vi "Log_ADAM_scan_table.vi"() -> ()   [LabVIEW 2022 SP3]
uses:
  ADAM Client/Sub VIs/ADAM Controls/Channel_State.ctl
  Anemometry/Anemometry Sub Vis/Globals/Constants_global.vi
  Anemometry/Anemometry Sub Vis/Globals/Preference_global.vi
  ADAM_Global.vi
  Anemometry/Anemometry Sub Vis/Globals/Meas_global.vi
  ADAM Client/Sub VIs/Channel_State_Control.ctl
panel:
  in  "Averaging time (Seconds)":dbl=60.0
  out "Current time":string
  out "Started Time":string
  in  "stop":bool
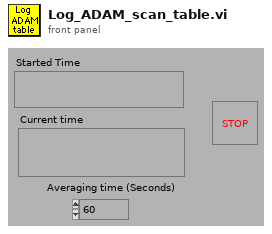
[diagram p1: front panel]
types:
  T1 = enum16{"On", "Off", "Always On", "Always Off", "Delete"}
  T2 = enum16{"Load ADAM setup from excel file", "Save ADAM setup to excel file"}
  T3 = typedef "Channel_State_Control.ctl" = enum16{"Channel Name", "Channel Name Starts with", "Main Address"}
  T4 = typedef "Channel_State.ctl" = enum16{"On", "Off", "Always On", "Always Off"}
  T5 = cluster{"second":i32, "minute":i32, "hour":i32, "day of month":i32, "month":i32, "year":i32, "day of week":i32, "day of year":i32, "is DST":i32}
  T6 = typedef "Client_State_Cluster.ctl" = cluster{"Client Name":string, "Traverse level State":T7, "People to Email":string[], "Next Contact Time":dbl}
  T7 = typedef "Traverse_Level_State.ctl" = enum16{"Running", "Complete"}
  T8 = typedef "Server_Control.ctl" = cluster{"Channel Name to control":string, "Channel sharing":enum16{"Channel Unshared", "Channel Shared by Rig", "Channel Shared by Group"}, "Default Value":dbl, "Client Array":string[], "Time Stamp":timestamp, "Do Not Reset":bool}
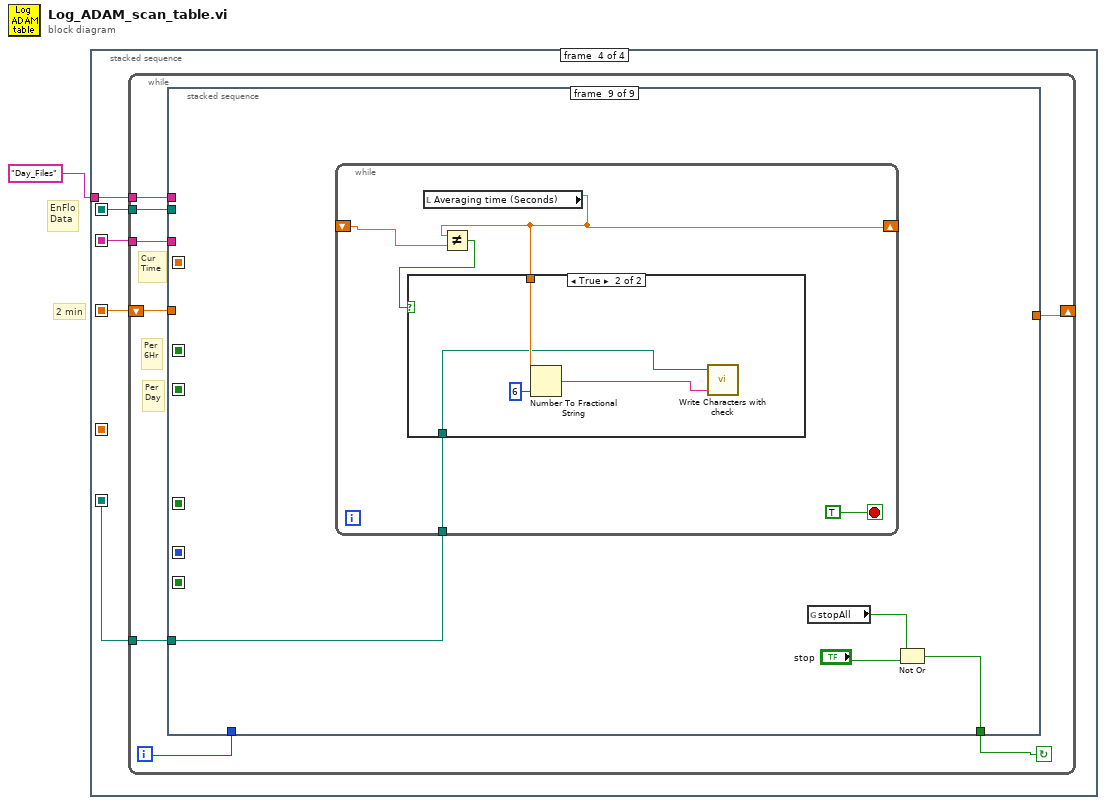
[diagram p0: block diagram]
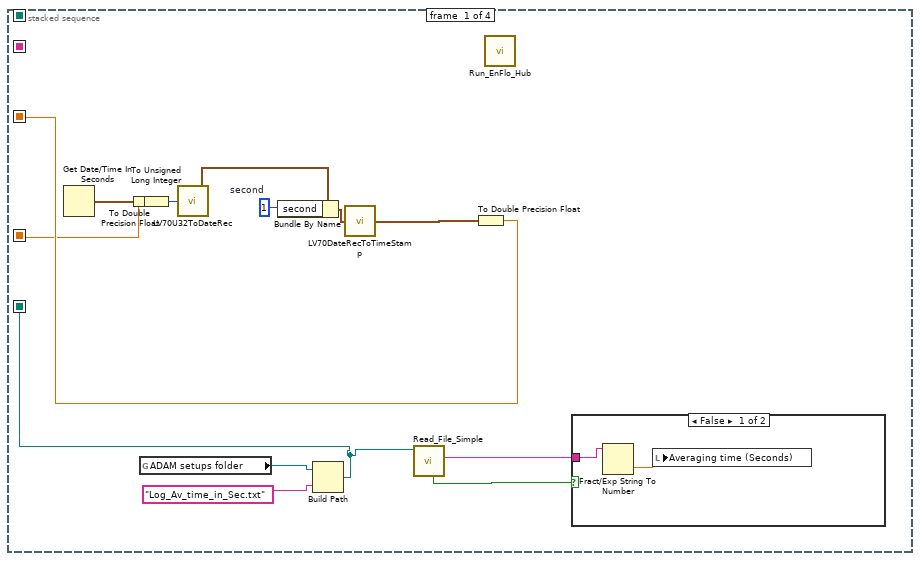
[diagram p2: hidden frame]
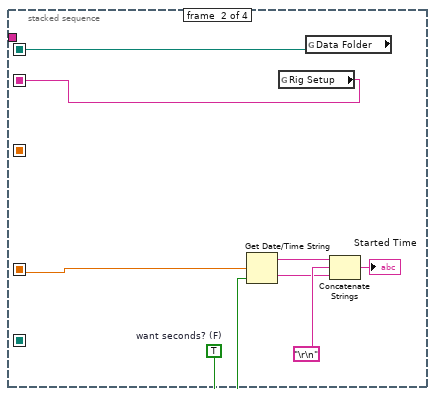
[diagram p4: hidden frame]
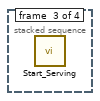
[diagram p5: hidden frame]
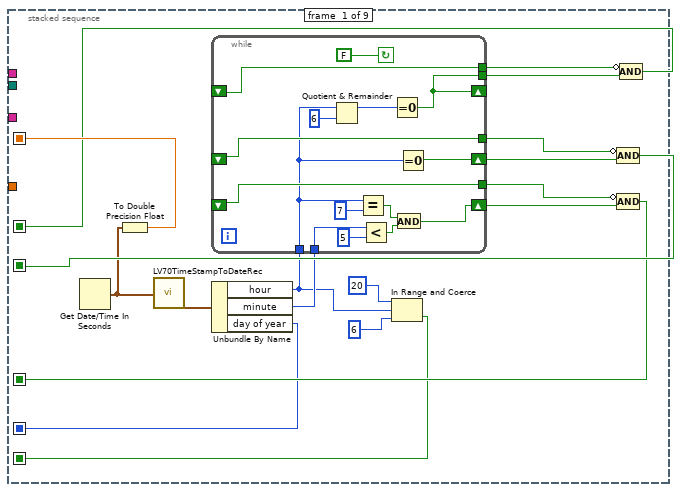
[diagram p6: hidden frame]
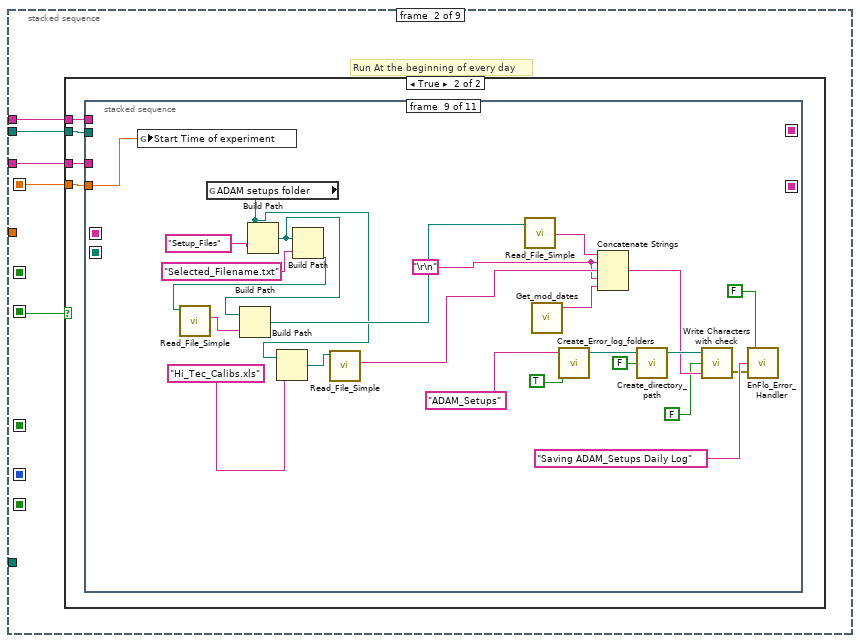
[diagram p7: hidden frame]
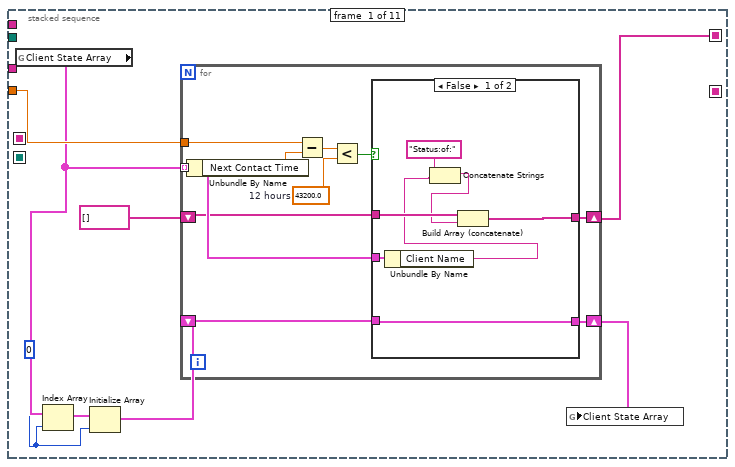
[diagram p9: hidden frame]
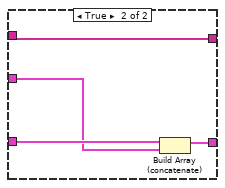
[diagram p10: hidden frame]
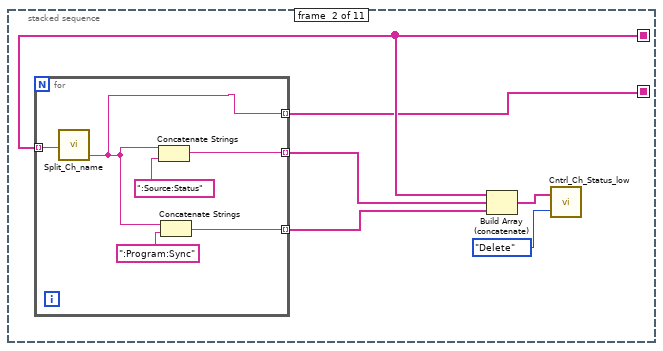
[diagram p11: hidden frame]
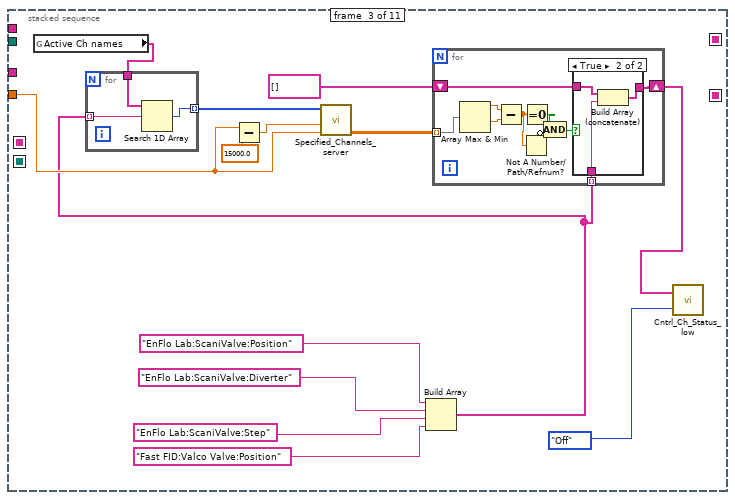
[diagram p12: hidden frame]
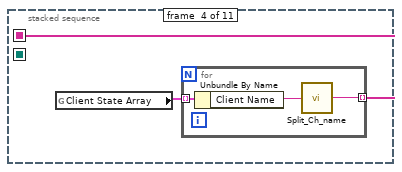
[diagram p14: hidden frame]
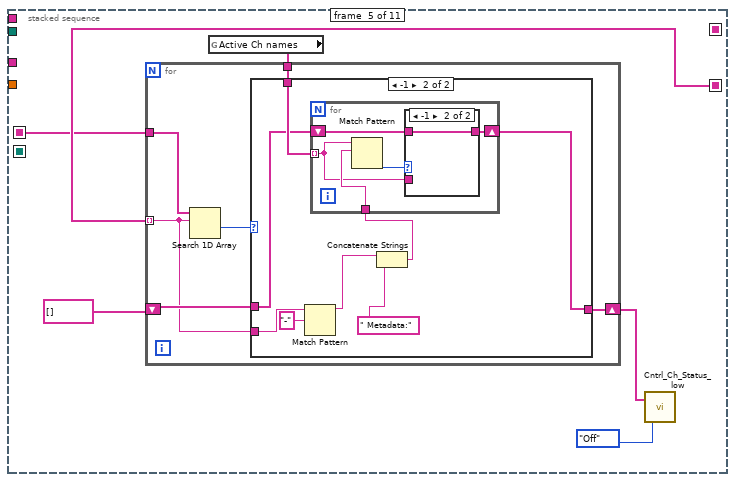
[diagram p15: hidden frame]
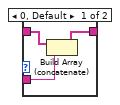
[diagram p17: hidden frame]
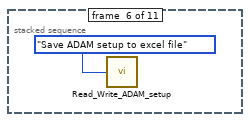
[diagram p18: hidden frame]
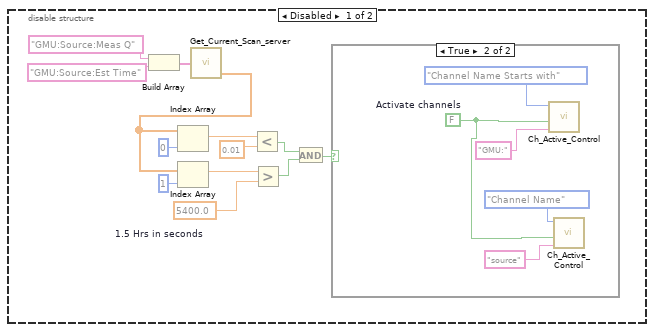
[diagram p20: hidden frame]
diagram:
  # "EnFlo\nData"
  # "2 min"
  n1 = stacked-sequence {
    seq-local: [w12 _ _ _] -> [_ _ _ w25]
    seq-local: [w11 _ _ _] -> [_ w24 _ _]
    seq-local: [_ w18 _ _] -> [_ _ _ w29]
    seq-local: [w4 _ _ _] -> [_ _ _ w27]
    seq-local: [_ w17 _ _] -> [_ _ _ w26]
    tunnel: "Day_Files" ("Input Element") -> [_ _ _ w28]
    frame #0 {
      w14 = 1  # second
      n2 = Get Date/Time In Seconds() -> (seconds since 1Jan1904=w8:timestamp)
      n3 = To Double Precision Float(number=w8) -> (double precision float=w11:dbl)
      n4 = global read "Constants_global.vi" "ADAM setups folder"() -> (w6:path)
      n5 = To Unsigned Long Integer(number=w11) -> (unsigned 32bit integer=w10:u32)
      n6 = call <vilib>:"LV70U32ToDateRec.vi"("Time"=w10) -> ("date time rec"=w9:T5)
      n7 = Bundle By Name(cluster=w9, "second"=w14) -> (w13:T5)
      n8 = Build Path(base path=w6, name or relative path="Log_Av_time_in_Sec.txt") -> (appended path=w4:path)
      n9 = call <vilib>:"LV70DateRecToTimeStamp.vi"("date time rec"=w13) -> ("Time Stamp"=w7:timestamp)
      n10 = call "Read_File_Simple.vi"("Filename"=w4) -> ("Error?"=w2:bool, "string"=w3:string)  [unwired: 2 in, 6 out]
      n11 = To Double Precision Float(number=w7) -> (double precision float=w12:dbl)
      n12 = call "Run_EnFlo_Hub.vi"() -> ()  [unwired: 1 in, 7 out]
      n13 = case shown="False" w2 {
        tunnel: w3 -> [w16 _]
        frame False {
          n14 = Fract/Exp String To Number(string=w16) -> (number=w15:dbl)  [unwired: 4 out]
          n15 = local write "Averaging time (Seconds)"(w15) -> ()
        }
        frame True {
        }
      }
    }
    frame #1 {
      w23 = TRUE  # want seconds? (F)
      n16 = Get Date/Time String(seconds (now)=w24, want seconds? (F)=w23) -> (date string=w21:string, time string=w20:string)  [unwired: 1 out]
      n17 = global read "Preference_global.vi" "Rig Setup"() -> (w17:string)
      n18 = global read "Constants_global.vi" "Data Folder"() -> (w18:path)
      n19 = Concatenate Strings(w21, "\r\n", w20) -> (→"Started Time":string)
    }
    frame #2 {
      n20 = call "Start_Serving.vi"() -> ()  [unwired: 1 out]
    }
    frame #3 {
      n21 = while {
        tunnel: w29 -> [w35]
        shift-left: w25 -> [w37]
        shift-right: [w36] -> _
        tunnel: w28 -> [w32]
        tunnel: w27 -> [w31]
        tunnel: w26 -> [w30]
        i -> [w34]
        stop <- w33 continue-if-true
        # "Per\n6Hr"
        # "Per\nDay"
        # "Cur\nTime"
        n22 = stacked-sequence {
          seq-local: [w48 _ _ _ _ _ _ _ _] -> [_ w75 _ _ _ _ _ _ _]
          seq-local: [w54 _ _ _ _ _ _ _ _] -> [_ w74 _ w307 _ w350 _ _ _]
          seq-local: [w51 _ _ _ _ _ _ _ _] -> [_ _ w274 _ _ _ _ _ _]
          seq-local: [w44 _ _ _ _ _ _ _ _] -> [_ _ _ w303 _ _ _ _ _]
          seq-local: [w42 _ _ _ _ _ _ _ _] -> [_ _ _ _ w327 _ _ _ _]
          seq-local: [w38 _ _ _ _ _ _ _ _] -> [_ _ _ _ w326 _ _ _ _]
          tunnel: [_ _ _ _ _ _ w362 _ _] -> w36
          tunnel: w37 -> [_ _ _ _ _ _ w363 _ _]
          tunnel: w35 -> [_ w73 _ w306 _ _ w370 _ _]
          tunnel: w34 -> [_ _ _ _ _ _ _ _ _]
          tunnel: [_ _ _ _ _ _ _ _ w401] -> w33
          tunnel: w32 -> [_ w72 _ w305 _ _ w360 _ _]
          tunnel: w31 -> [_ _ _ _ _ _ _ _ w400]
          tunnel: w30 -> [_ w71 _ w304 _ _ w364 _ _]
          frame #0 {
            n23 = Get Date/Time In Seconds() -> (seconds since 1Jan1904=w47:timestamp)
            n24 = To Double Precision Float(number=w47) -> (double precision float=w54:dbl)
            n25 = call <vilib>:"LV70TimeStampToDateRec.vi"("time stamp"=w47) -> ("date time rec"=w55:T5)
            n26 = Unbundle By Name(w55) -> ("hour"=w41:i32, "minute"=w43:i32, "day of year"=w42:i32)
            n27 = while {
              tunnel: [w65] -> w49
              shift-left: _ -> [w65]
              shift-right: [w66] -> w50
              tunnel: [w67] -> w52
              tunnel: [w68] -> w53
              tunnel: w41 -> [w62]
              shift-left: _ -> [w67]
              shift-right: [w68] -> _
              tunnel: [w63] -> w46
              shift-right: [w56] -> w45
              shift-left: _ -> [w63]
              tunnel: w43 -> [w60]
              stop <- FALSE continue-if-true
              n28 = Quotient & Remainder(x=w62, y=6) -> (x-y*floor(x/y)=w69:i32)  [unwired: 1 out]
              n29 = Equal?(x=w62, y=7) -> (x = y?=w57:bool)
              n30 = Less?(x=w60, y=5) -> (x < y?=w58:bool)
              n31 = Equal To 0?(x=w69) -> (x = 0?=w68:bool)
              n32 = And(x=w57, y=w58) -> (x .and. y?=w56:bool)
              n33 = Equal To 0?(x=w62) -> (x = 0?=w66:bool)
            }
            n34 = In Range and Coerce(upper limit=20, x=w41, lower limit=6) -> (In Range?=w38:bool)  [unwired: 1 out]
            n35 = Compound Arithmetic op=AND(invert w49, w50) -> (w48:bool)
            n36 = Compound Arithmetic op=AND(invert w46, w45) -> (w44:bool)
            n37 = Compound Arithmetic op=AND(invert w52, w53) -> (w51:bool)
          }
          frame #1 {
            # "Run At the beginning of every day"
            n38 = case shown="True" w75 {
              tunnel: w74 -> [_ w79]
              tunnel: w73 -> [_ w78]
              tunnel: w72 -> [_ w77]
              tunnel: w71 -> [_ w76]
              frame False {
              }
              frame True {
                n39 = stacked-sequence {
                  seq-local: [w80 _ _ _ _ _ _ _ _ _ _] -> [_ w114 _ _ _ _ _ w207 _ _ _]
                  seq-local: [_ w110 _ _ _ _ _ _ _ _ _] -> [_ _ _ _ w162 _ _ _ _ _ _]
                  seq-local: [_ _ _ w152 _ _ _ _ _ _ _] -> [_ _ _ _ w159 _ _ _ _ _ _]
                  seq-local: [_ _ _ _ _ _ _ _ _ w260 _] -> [_ _ _ _ _ _ _ _ _ _ w264]
                  tunnel: w79 -> [w87 _ w131 _ _ _ _ _ w258 _ w265]
                  tunnel: w78 -> [_ _ _ _ _ _ _ _ _ _ _]
                  tunnel: w77 -> [_ _ _ _ _ _ _ _ _ _ _]
                  tunnel: w76 -> [_ _ _ _ _ _ _ _ _ _ _]
                  frame #0 {
                    w85 = 0 ("Index")
                    n40 = global read "ADAM_Global.vi" "Client State Array"() -> (w86:T6[])
                    n41 = Index Array(array=w86, index=w85) -> (element=w84:T6)
                    n42 = Initialize Array(w84, w85) -> (w83:T6[])
                    n43 = for {
                      tunnel: w86 -> [w90] mode=indexing
                      shift-right: [w91] -> w82
                      shift-left: w83 -> [w92]
                      tunnel: w87 -> [w97]
                      shift-right: [w88] -> w80
                      shift-left: string[] [] -> [w89]
                      w94 = 43200.0  # 12 hours
                      n44 = Unbundle By Name(w90) -> ("Next Contact Time"=w96:dbl)
                      n45 = Subtract(x=w97, y=w96) -> (x-y=w95:dbl)
                      n46 = Less?(x=w95, y=w94) -> (x < y?=w93:bool)
                      n47 = case shown="False" w93 {
                        tunnel: w92 -> [w104 w108]
                        tunnel: [w104 w107] -> w91
                        tunnel: w90 -> [w103 w106]
                        tunnel: w89 -> [w102 w105]
                        tunnel: [w101 w105] -> w88
                        frame False {
                          n48 = Unbundle By Name(w103) -> ("Client Name"=w99:string)
                          n49 = Concatenate Strings("Status:of:", w99) -> (w98:string)
                          n50 = Build Array (concatenate)(w102, w98) -> (w101:string[])
                        }
                        frame True {
                          n51 = Build Array (concatenate)(w108, w106) -> (w107:T6[])
                        }
                      }
                    }
                    n52 = global write "ADAM_Global.vi" "Client State Array"(w82) -> ()
                  }
                  frame #1 {
                    n53 = for {
                      tunnel: w114 -> [w120] mode=indexing
                      tunnel: [w117] -> w112 mode=indexing
                      tunnel: [w116] -> w111 mode=indexing
                      tunnel: [w115] -> w110 mode=indexing
                      n54 = call "Split_Ch_name.vi"("Ch name"=w120) -> ("Low level"=w115:string)  [unwired: 2 out]
                      n55 = Concatenate Strings(w115, ":Source:Status") -> (w117:string)
                      n56 = Concatenate Strings(w115, ":Program:Sync") -> (w116:string)
                    }
                    n57 = Build Array (concatenate)(w114, w112, w111) -> (w113:string[])
                    n58 = call "Cntrl_Ch_Status_low.vi"("Mode"=T1."Delete", "Channel names"=w113) -> ()  [unwired: 1 out]
                  }
                  frame #2 {
                    n59 = global read "ADAM_Global.vi" "Active Ch names"() -> (w134:string[])
                    n60 = Subtract(x=w131, y=15000.0) -> (x-y=w129:dbl)
                    n61 = Build Array("EnFlo Lab:ScaniValve:Position", "EnFlo Lab:ScaniValve:Diverter", "EnFlo Lab:ScaniValve:Step", "Fast FID:Valco Valve:Position") -> (w127:string[])
                    n62 = for {
                      tunnel: w134 -> [w151]
                      tunnel: w127 -> [w150] mode=indexing
                      tunnel: [w149] -> w132 mode=indexing
                      n63 = Search 1D Array(1D array=w151, element=w150) -> (index of element=w149:i32)  [unwired: 1 out]
                    }
                    n64 = call "Specified_Channels_server.vi"("End time"=w131, "Start time"=w129, "Requested channels"=w132) -> ("Output array"=w128:dbl[][])  [unwired: 2 in, 4 out]
                    n65 = for {
                      tunnel: w128 -> [w141] mode=indexing
                      shift-right: [w142] -> w122
                      shift-left: string[] [] -> [w136]
                      tunnel: w127 -> [w137] mode=indexing
                      n66 = Array Max & Min(array=w141) -> (max value=w144:dbl, min value=w143:dbl)  [unwired: 2 out]
                      n67 = Subtract(x=w144, y=w143) -> (x-y=w140:dbl)
                      n68 = Not A Number/Path/Refnum?(number/path/refnum=w140) -> (NaN/Path/Refnum?=w138:bool)
                      n69 = Equal To 0?(x=w140) -> (x = 0?=w135:bool)
                      n70 = Compound Arithmetic op=AND(w135, invert w138) -> (w139:bool)
                      n71 = case shown="True" w139 {
                        tunnel: [w145 w148] -> w142
                        tunnel: w137 -> [_ w147]
                        tunnel: w136 -> [w145 w146]
                        frame False {
                        }
                        frame True {
                          n72 = Build Array (concatenate)(w146, w147) -> (w148:string[])
                        }
                      }
                    }
                    n73 = call "Cntrl_Ch_Status_low.vi"("Mode"=T1."Off", "Channel names"=w122) -> ()  [unwired: 1 out]
                  }
                  frame #3 {
                    n74 = global read "ADAM_Global.vi" "Client State Array"() -> (w153:T6[])
                    n75 = for {
                      tunnel: w153 -> [w156] mode=indexing
                      tunnel: [w154] -> w152 mode=indexing
                      n76 = Unbundle By Name(w156) -> ("Client Name"=w155:string)
                      n77 = call "Split_Ch_name.vi"("Ch name"=w155) -> ("Middle"=w154:string)  [unwired: 2 out]
                    }
                  }
                  frame #4 {
                    n78 = global read "ADAM_Global.vi" "Active Ch names"() -> (w160:string[])
                    n79 = for {
                      tunnel: w162 -> [w163] mode=indexing
                      shift-right: [w166] -> w158
                      shift-left: string[] [] -> [w167]
                      tunnel: w160 -> [w165]
                      tunnel: w159 -> [w164]
                      n80 = Search 1D Array(1D array=w164, element=w163) -> (index of element=w168:i32)  [unwired: 1 out]
                      n81 = case shown="-1" w168 {
                        tunnel: w167 -> [w169 w175]
                        tunnel: [w169 w174] -> w166
                        tunnel: w163 -> [_ w170]
                        tunnel: w165 -> [_ w176]
                        frame 0, Default {
                        }
                        frame -1 {
                          n82 = Match Pattern(string=w170, regular expression="-") -> (before substring=w171:string)  [unwired: 4 out]
                          n83 = Concatenate Strings(w171, " Metadata:" ("Substring")) -> (w173:string)
                          n84 = for {
                            shift-right: [w180] -> w174
                            shift-left: w175 -> [w181]
                            tunnel: w173 -> [w179]
                            tunnel: w176 -> [w178] mode=indexing
                            n85 = Match Pattern(string=w178, regular expression=w179) -> (offset past match=w182:i32)  [unwired: 4 out]
                            n86 = case shown="-1" w182 {
                              tunnel: w181 -> [w184 w186]
                              tunnel: [w183 w186] -> w180
                              tunnel: w178 -> [w185 _]
                              frame 0, Default {
                                n87 = Build Array (concatenate)(w184, w185) -> (w183:string[])
                              }
                              frame -1 {
                              }
                            }
                          }
                        }
                      }
                    }
                    n88 = call "Cntrl_Ch_Status_low.vi"("Mode"=T1."Off", "Channel names"=w158) -> ()  [unwired: 1 out]
                  }
                  frame #5 {
                    n89 = call "Read_Write_ADAM_setup.vi"("Mode"=T2."Save ADAM setup to excel file") -> ()  [unwired: 4 out]
                  }
                  frame #6 {
                    n90 = disable-structure shown="Enabled" {
                      frame Disabled {
                        w191 = 5400.0  # 1.5 Hrs in seconds
                        n91 = Build Array("GMU:Source:Meas Q", "GMU:Source:Est Time") -> (w198:string[])
                        n92 = call "Get_Current_Scan_server.vi"("Desired Channels"=w198) -> ("Numerical Values"=w193:dbl[])  [unwired: 2 out]
                        n93 = Index Array(array=w193, index=0 ("Index")) -> (element=w195:dbl)
                        n94 = Index Array(array=w193, index=1 ("Index")) -> (element=w192:dbl)
                        n95 = Less?(x=w195, y=0.01) -> (x < y?=w189:bool)
                        n96 = Greater?(x=w192, y=w191) -> (0:w190:bool)
                        n97 = And(x=w189, y=w190) -> (x .and. y?=w188:bool)
                        n98 = case shown="True" w188 {
                          frame False {
                          }
                          frame True {
                            w202 = FALSE  # Activate channels
                            n99 = call "Ch_Active_Control.vi"("Match"="GMU:", "Activate Channels?"=w202, "Control on"=Channel_State_Control."Channel Name Starts with") -> ()  [unwired: 1 in, 2 out]
                            n100 = call "Ch_Active_Control.vi"("Match"="source", "Activate Channels?"=w202, "Control on"=Channel_State_Control."Channel Name") -> ()  [unwired: 1 in, 2 out]
                          }
                        }
                      }
                      frame Enabled {
                      }
                    }
                  }
                  frame #7 {
                    w211 = 0 ("Index")
                    n101 = global read "ADAM_Global.vi" "Server Control Array"() -> (w208:T8[])
                    n102 = Index Array(array=w208, index=w211) -> (element=w210:T8)
                    n103 = Initialize Array(w210, w211) -> (w209:T8[])
                    n104 = for {
                      tunnel: w208 -> [w213] mode=indexing
                      shift-right: [w218] -> w206
                      shift-left: w209 -> [w219]
                      tunnel: w207 -> [w217]
                      n105 = Unbundle By Name(w213) -> ("Client Array"=w216:string[])
                      n106 = for {
                        tunnel: w217 -> [w224]
                        tunnel: w216 -> [w222] mode=indexing
                        shift-right: [w220] -> w212
                        shift-left: string[] [] -> [w221]
                        n107 = Search 1D Array(1D array=w224, element=w222) -> (index of element=w223:i32)  [unwired: 1 out]
                        n108 = case shown="0, Default" w223 {
                          tunnel: w222 -> [_ w228]
                          tunnel: w221 -> [w225 w227]
                          tunnel: [w225 w226] -> w220
                          frame 0, Default {
                          }
                          frame -1 {
                            n109 = Build Array (concatenate)(w227, w228) -> (w226:string[])
                          }
                        }
                      }
                      n110 = Array Size(array=w212) -> (size(s)=w214:i32)
                      n111 = case shown="1, Default" w214 {
                        tunnel: w219 -> [w229 w233]
                        tunnel: [w229 w234] -> w218
                        tunnel: w213 -> [_ w232]
                        tunnel: w212 -> [_ w231]
                        frame 0 {
                        }
                        frame 1, Default {
                          n112 = Bundle By Name(cluster=w232, "Client Array"=w231) -> (w230:T8)
                          n113 = Build Array (concatenate)(w233, w230) -> (w234:T8[])
                        }
                      }
                    }
                    n114 = global write "ADAM_Global.vi" "Server Control Array"(w206) -> ()
                  }
                  frame #8 {
                    w246 = "\r\n"
                    n115 = global write "Meas_global.vi" "Start Time of experiment"(w258) -> ()
                    n116 = global read "Constants_global.vi" "ADAM setups folder"() -> (w249:path)
                    n117 = Build Path(base path=w249, name or relative path="Setup_Files") -> (appended path=w253:path)
                    n118 = Build Path(base path=w249, name or relative path="Hi_Tec_Calibs.xls") -> (appended path=w248:path)
                    n119 = Build Path(base path=w253, name or relative path="Selected_Filename.txt" ("Substring")) -> (appended path=w255:path)
                    n120 = call "Read_File_Simple.vi"("Filename"=w255) -> ("string"=w254:string)  [unwired: 2 in, 7 out]
                    n121 = Build Path(base path=w253, name or relative path=w254) -> (appended path=w252:path)
                    n122 = call "Read_File_Simple.vi"("Filename"=w248) -> ("string"=w247:string)  [unwired: 2 in, 7 out]
                    n123 = call "Read_File_Simple.vi"("Filename"=w252) -> ("string"=w251:string)  [unwired: 2 in, 7 out]
                    n124 = call "Get_mod_dates.vi"() -> ("Output string"=w245:string)  [unwired: 1 in, 4 out]
                    n125 = call "Create_Error_log_folders.vi"("Log Filename"="ADAM_Setups" ("Substring"), "Per Day Log File?"=TRUE) -> ("Local Log File"=w242:path)  [unwired: 4 in, 1 out]
                    n126 = Concatenate Strings(w251, w246, w247, w246, w245) -> (w237:string)
                    n127 = call "Create_directory_path.vi"("Dialog Box"=FALSE, "Path name"=w242) -> ("Path name Out"=w238:path)  [unwired: 1 in, 1 out]
                    n128 = call "Write Characters with check.vi"("String to Write"=w237, "Call EnFlo Error Handler?"=FALSE, "file (use dialog)"=w238) -> ("error out"=w236:errorcluster)  [unwired: 1 in]
                    n129 = call "EnFlo_Error_Handler.vi"("error in (no error)"=w236, "Error Type"="Saving ADAM_Setups Daily Log", "Dialog Box (F)"=FALSE ("Dialog Box (T)")) -> ()  [unwired: 1 in, 2 out]
                  }
                  frame #9 {
                    n130 = global read "Constants_global.vi" "Data Folder Local"() -> (w261:path)
                    n131 = Build Path(base path=w261, name or relative path="Results_Summary_files") -> (appended path=w260:path)
                  }
                  frame #10 {
                    # "If the summary files are more than 60 days old delete them"
                    n132 = To Unsigned Long Integer(number=w265) -> (unsigned 32bit integer=w262:u32)
                    n133 = call "Get_folder_and_filenames.vi"("file path (dialog if empty)"=w264) -> ("Files"=w263:path[])  [unwired: 1 out]
                    n134 = for {
                      tunnel: w263 -> [w267] mode=indexing
                      tunnel: w262 -> [w272]
                      # "60 days in seconds"
                      n135 = File/Directory Info(path=w267) -> (last mod=w266:timestamp)  [unwired: 1 in, 6 out]
                      n136 = To Unsigned Long Integer(number=w266) -> (unsigned 32bit integer=w271:u32)
                      n137 = Subtract(x=w272, y=w271) -> (x-y=w270:u32)
                      n138 = Greater?(x=w270, y=u32 5184000) -> (0:w268:bool)
                      n139 = case shown="True" w268 {
                        tunnel: w267 -> [_ w273]
                        frame False {
                        }
                        frame True {
                          n140 = Delete(path (use dialog)=w273) -> ()  [unwired: 1 in, 6 out]
                        }
                      }
                    }
                  }
                }
              }
            }
          }
          frame #2 {
            # "Do every 6 Hours"
            n141 = case shown="True" w274 {
              frame False {
              }
              frame True {
                n142 = Build Array("EnFlo_Tunnel:Bus Bar + Heaters:Enable") -> (w280:string[])
                n143 = call "Get_Current_Scan_server.vi"("Desired Channels"=w280) -> ("Numerical Values"=w279:dbl[])  [unwired: 2 out]
                n144 = Index Array(array=w279, index=0) -> (element=w277:dbl)
                n145 = Less?(x=w277, y=0.5) -> (x < y?=w275:bool)
                n146 = case shown="True" w275 {
                  frame False {
                  }
                  frame True {
                    w286 = "EnFlo_Tunnel:Setpo"
                    n147 = global read "ADAM_Global.vi" "Active Ch names"() -> (w284:string[])
                    n148 = String Length(string=w286) -> (length=w285:i32)
                    n149 = for {
                      shift-right: [w294] -> w283
                      shift-left: string[] [] -> [w296]
                      tunnel: w284 -> [w295] mode=indexing
                      tunnel: w285 -> [w298]
                      tunnel: w286 -> [w297]
                      tunnel: "EnFlo_Tunnel:Power" -> [w292]
                      n150 = String Subset(string=w295, length (rest)=w298) -> (substring=w293:string)  [unwired: 1 out]
                      n151 = Equal?(x=w293, y=w297) -> (x = y?=w290:bool)
                      n152 = Equal?(x=w293, y=w292) -> (x = y?=w291:bool)
                      n153 = Or(x=w290, y=w291) -> (x .or. y?=w289:bool)
                      n154 = case shown="True" w289 {
                        tunnel: w296 -> [w299 w302]
                        tunnel: w295 -> [_ w301]
                        tunnel: [w299 w300] -> w294
                        frame False {
                        }
                        frame True {
                          n155 = Build Array (concatenate)(w302, w301) -> (w300:string[])
                        }
                      }
                    }
                    n156 = call "Adam_Ch_on_off.vi"("Ch State"=Channel_State."Off", "ADAM Ch Names"=w283) -> ()  [unwired: 1 out]
                  }
                }
              }
            }
          }
          frame #3 {
            # "At 7am every day"
            n157 = case shown="True" w303 {
              tunnel: w307 -> [_ w311]
              tunnel: w306 -> [_ w310]
              tunnel: w305 -> [_ w309]
              tunnel: w304 -> [_ w308]
              frame False {
              }
              frame True {
                n158 = stacked-sequence {
                  seq-local: [w320 _] -> [_ w325]
                  tunnel: w311 -> [w323 _]
                  tunnel: w310 -> [w314 _]
                  tunnel: w309 -> [w318 _]
                  tunnel: w308 -> [w315 _]
                  frame #0 {
                    n159 = Subtract(x=w323, y=36000.0) -> (x-y=w322:dbl)
                    n160 = call "Sec_to_date_filename.vi"("ss1904"=w322) -> ("YYYY"=w319:string, "mm-YYYY"=w313:string, "DD-mm-YYYY"=w312:string)  [unwired: 5 in, 7 out]
                    n161 = Concatenate Strings(w312, ".xls" ("string")) -> (w316:string)
                    n162 = Build Array(w319, w315, w318, w313, w316) -> (w321:string[])
                    n163 = call "Build_Pathname.vi"("PathElements"=w321, "PathnameIn"=w314) -> ("AppendedPath"=w320:path)
                  }
                  frame #1 {
                    # "This VI emails a summary of all the server errors that occured Yesterday"
                    n164 = call "Adam_server_messages.vi"("Filename"=w325) -> ()  [unwired: 1 out]
                  }
                }
              }
            }
          }
          frame #4 {
            # "Backup             \"EnFlo_Data_Current\"        to     \"EnFlo_Data\""
            n165 = case shown="True" w326 {
              tunnel: w327 -> [_ w328]
              frame False {
              }
              frame True {
                n166 = while {
                  shift-right: [w334] -> _
                  shift-left: _ -> [w331]
                  tunnel: w328 -> [w330]
                  stop <- TRUE stop-if-true
                  n167 = Greater Than 0?(x=w331) -> (x > 0?=w332:bool)
                  n168 = Select(t=w331, s=w332, f=w330) -> (s? t:f=w329:i32)
                  n169 = Equal?(x=w329, y=w330) -> (x = y?=w333:bool)
                  n170 = case shown="False" w333 {
                    tunnel: [w338 w349] -> w334
                    tunnel: w330 -> [w337 _]
                    tunnel: w329 -> [w336 w349]
                    frame False {
                      n171 = Build Array("EnFlo_Tunnel:Heater:Enable") -> (w343:string[])
                      n172 = call "Get_Current_Scan_server.vi"("Desired Channels"=w343) -> ("Numerical Values"=w342:dbl[])  [unwired: 2 out]
                      n173 = Index Array(array=w342) -> (element=w341:dbl)  [unwired: 1 in]
                      n174 = Greater?(x=w341, y=0.5) -> (0:w339:bool)
                      n175 = case shown="False" w339 {
                        tunnel: [w345 w348] -> w338
                        tunnel: w337 -> [w345 _]
                        tunnel: w336 -> [_ w348]
                        frame False {
                          n176 = call "Robocopy Current Backup.vi"("Dest. drive root"=path "S:/Research/EnFlo_Data", "Source drive root"=path "S:/Research/EnFlo_Data_Current") -> ()  [unwired: 4 in, 3 out]
                        }
                        frame True {
                        }
                      }
                    }
                    frame True {
                    }
                  }
                }
              }
            }
          }
          frame #5 {
            n177 = call "EnFlo_Seeder_Control.vi"("Current Time (s)"=w350) -> ()
            n178 = Wait (ms)(milliseconds to wait=u32 1000 ("milliseconds to Wait")) -> ()  [unwired: 1 out]
          }
          frame #6 {
            n179 = global read "ADAM_Global.vi" "Scan Index"() -> (w353:i32)
            n180 = Divide(x="Averaging time (Seconds)", y=60.0) -> (x/y=w368:dbl)
            n181 = Divide(x="Averaging time (Seconds)", y=2.0) -> (x/y=w365:dbl)
            n182 = feedback #1() -> (w354:i32)  [unwired: 1 in]
            n183 = Add(x=w365, y=w363) -> (x+y=w361:dbl)
            n184 = call "Sec_to_date_filename.vi"("ss1904"=w361) -> ("YYYY"=w372:string, "mm-YYYY"=w352:string, "DD-mm-YYYY"=w357:string)  [unwired: 5 in, 7 out]
            n185 = Concatenate Strings(w357, ".xls" ("string")) -> (w359:string)
            n186 = Not Equal?(x=w354, y=w353) -> (x != y?=w356:bool)
            n187 = Build Array(w372, w364, w360, w352, w359) -> (w371:string[])
            n188 = call "Time_elapsed.vi"("End of previous average in"=w363, "New Scan Index?"=w356, "Averaging time (mins)"=w368) -> ("End of previous average out"=w362:dbl, "End of period"=w374:dbl, "Start of period"=w375:dbl, "Take new reading?"=w373:bool)  [unwired: 1 in]
            n189 = case shown="True" w373 {
              tunnel: w374 -> [_ w381]
              tunnel: w375 -> [_ w382]
              tunnel: w370 -> [_ w380]
              tunnel: w371 -> [_ w379]
              tunnel: [w376 w378] -> w355
              tunnel: w354 -> [w376 _]
              tunnel: w353 -> [_ w377]
              frame False {
              }
              frame True {
                n190 = stacked-sequence {
                  tunnel: w382 -> [w391 _]
                  tunnel: w381 -> [w390 _]
                  tunnel: w380 -> [w383 _]
                  tunnel: w379 -> [w386 _]
                  tunnel: [_ w392] -> w378
                  tunnel: w377 -> [_ w392]
                  frame #0 {
                    n191 = global read "ADAM_Global.vi" "2 Min average comment"() -> (w389:string)
                    n192 = global read "Meas_global.vi" "Error Messages"() -> (w388:string)
                    n193 = call "Build_Pathname.vi"("PathElements"=w386, "PathnameIn"=w383) -> ("AppendedPath"=w385:path)
                    n194 = call "Create_directory_path.vi"("Path name"=w385) -> ("Path name Out"=w384:path)  [unwired: 2 in, 1 out]
                    n195 = Concatenate Strings(w389, w388) -> (w387:string)
                    n196 = call "Write_to_log_file.vi"("User added comment"=w387, "End time"=w390, "Start time"=w391, "Folder/file"=w384) -> ()  [unwired: 5 in, 3 out]
                  }
                  frame #1 {
                    w393 = ""
                    n197 = global write "ADAM_Global.vi" "2 Min average comment"(w393) -> ()
                    n198 = global write "Meas_global.vi" "Error Messages"(w393) -> ()
                  }
                }
              }
            }
            n199 = feedback-in #1(w355) -> ()
          }
          frame #7 {
            w398 = TRUE  # want seconds? (F)
            n200 = Get Date/Time String(want seconds? (F)=w398) -> (date string=w396:string, time string=w395:string)  [unwired: 2 out]
            n201 = Concatenate Strings(w396, "\r\n", w395) -> (→"Current time":string)
          }
          frame #8 {
            n202 = while {
              shift-right: [w403] -> _
              shift-left: _ -> [w407]
              tunnel: w400 -> [w404]
              stop <- TRUE stop-if-true
              n203 = local read "Averaging time (Seconds)"() -> (w403:dbl)
              n204 = Not Equal?(x=w403, y=w407) -> (x != y?=w405:bool)
              n205 = case shown="True" w405 {
                tunnel: w404 -> [_ w409]
                tunnel: w403 -> [_ w410]
                frame False {
                }
                frame True {
                  n206 = Number To Fractional String(number=w410, precision (6)=i16 6) -> (F-format string=w408:string)  [unwired: 2 out]
                  n207 = call "Write Characters with check.vi"("String to Write"=w408, "file (use dialog)"=w409) -> ()  [unwired: 2 in, 1 out]
                }
              }
            }
            n208 = global read "ADAM_Global.vi" "stopAll"() -> (w399:bool)
            n209 = Not Or(1:"stop", 2:w399) -> (0:w401:bool)
          }
        }
      }
    }
  }
